vi "Teleop.vi"(10 "Match Info":T1={"Autonomous Elapsed Seconds"=0.0, "TeleOp Elapsed Seconds"=0.0, "Disabled Elapsed Seconds"=0.0, "Visited Autonomous"=FALSE, "Visited TeleOp"=FALSE, "Visited Disabled"=FALSE, "Autonomous Settings"={"Autonomous Style"=enum."Independent", "VI Refnum"=refnum}}, 11 "Call Context":T2) -> ()   [LabVIEW 2012]
doc: "This VI is called for each TeleOp packet received from the DS where the robot is not disabled. It is often used to read from the joysticks and update I/O or to update setpoints for timed control loops. It should complete and return within 20 milliseconds or it may miss DS packets."
uses:
  Robot Global Data.vi
  <vilib>/Rock Robotics/WPI/RobotDrive/WPI_RobotDriveMotorSelectorEnum.ctl
  <vilib>/Rock Robotics/WPI/Solenoid/WPI_SolenoidValue.ctl
  <vilib>/Rock Robotics/WPI/Solenoid/WPI_SolenoidSetEnum.vi
  <vilib>/Rock Robotics/WPI/RobotDrive/WPI_RobotDriveMecanumDrive_Cartesian.vi
  <vilib>/Rock Robotics/WPI/DriverStation/WPI_DriverStationMatch Info.ctl
  <vilib>/Rock Robotics/WPI/DriverStation/WPI_DriverStationDerivedRobotMode.ctl
panel:
  out "Frount/Rear drive speed":dbl=0.33
  out "MECH X/Y Speed":dbl=1.0
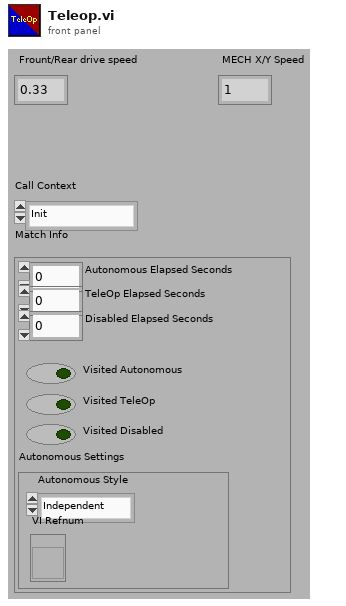
[diagram p1: front panel]
types:
  T1 = typedef "WPI_DriverStationMatch Info.ctl" = cluster{"Autonomous Elapsed Seconds":dbl, "TeleOp Elapsed Seconds":dbl, "Disabled Elapsed Seconds":dbl, "Visited Autonomous":bool, "Visited TeleOp":bool, "Visited Disabled":bool, "Autonomous Settings":cluster{"Autonomous Style":enum16{"Iterative", "Independent"}, "VI Refnum":refnum<vi>}}
  T2 = typedef "WPI_DriverStationDerivedRobotMode.ctl" = enum16{"Init", "Execute", "Stop"}
  T3 = typedef "WPI_SolenoidValue.ctl" = enum16{"Off", "On", "Forward", "Reverse"}
  T4 = typedef "WPI_JoystickDevRef.ctl" = cluster{"Device":T5}
  T5 = typedef "WPI_JoystickDeviceEnum.ctl" = enum16{"USB 1", "USB 2", "USB 3", "USB 4", "Kinect 1", "Kinect 2"}
  T6 = typedef "WPI_JoystickButtonState.ctl" = cluster{"Button 1":bool, "Button 2":bool, "Button 3":bool, "Button 4":bool, "Button 5":bool, "Button 6":bool, "Button 7":bool, "Button 8":bool, "Button 9":bool, "Button 10":bool, "Button 11":bool, "Button 12":bool}
  T7 = cluster{"axis 1 (x)":dbl, "axis 2 (y)":dbl, "axis 3 (throttle)":dbl, "axis 4":dbl, "axis 5":dbl, "axis 6":dbl}
  T8 = typedef "WPI_RobotDriveDevRef.ctl" = cluster{"DevStatus":errorcluster, "Motors[]":T9[], "Square Inputs":bool, "Max Output":dbl, "Isochronous":bool}
  T9 = typedef "WPI_MotorControlDeviceRef.ctl" = cluster{"DeviceStatus":errorcluster, "Type":enum16{"PWM", "CAN"}, "PWM":cluster{"Digital Module":T10, "PWM Channel":T11, "DeadBand":T12}, "CAN":cluster{"Device Number":u8, "Control Mode":T13, "Semaphore":T14, "Max Vout":dbl}, "Invert":bool, "TransformRef":T15, "InvTransformRef":T15}
  T10 = typedef "FPGA_TypedefDigitalModule.ctl" = enum16{"Digital Module 1", "Digital Module 2"}
  T11 = typedef "FPGA_DIOPWMChannel.ctl" = enum8{"PWM 1", "PWM 2", "PWM 3", "PWM 4", "PWM 5", "PWM 6", "PWM 7", "PWM 8", "PWM 9", "PWM 10", "Invalid"}
  T12 = typedef "WPI_PWMDeadband.ctl" = cluster{"Name":string, "maxPositivePwm":i32, "minPositivePwm":i32, "centerPwm":i32, "maxNegativePwm":i32, "minNegativePwm":i32, "angularRange":u16}
  T13 = typedef "WPI_CANJaguar_ControlMode.ctl" = enum8{"Percent VBus", "Current", "Speed", "Position", "Voltage"}
  T14 = typedef "Semaphore RefNum" = refnum<k1>
  T15 = typedef "WPI_PWMTransform_ConPane.ctl" = refnum<vi>
  T16 = typedef "WPI_RobotDriveMotorSelectorEnum.ctl" = enum16{"Rear Left Motor", "Rear Right Motor", "Front Left Motor", "Front Right Motor"}
  T17 = typedef "WPI_DigitalInputDevRef.ctl" = cluster{"DevStatus":errorcluster, "DIO Channel":T18, "Digital Module":T10}
  T18 = typedef "FPGA_DIOChannel.ctl" = enum8{"DIO 1", "DIO 2", "DIO 3", "DIO 4", "DIO 5", "DIO 6", "DIO 7", "DIO 8", "DIO 9", "DIO 10", "DIO 11", "DIO 12", "DIO 13", "DIO 14", "Invalid"}
  T19 = typedef "WPI_SolenoidDevRef.ctl" = cluster{"DevStatus":errorcluster, "Solenoid Module":T20, "Forward Solenoid Channel":T21, "Reverse Solenoid Channel":T21}
  T20 = typedef "FPGA_TypedefSolenoidModule.ctl" = enum16{"Solenoid Module 1", "Solenoid Module 2"}
  T21 = typedef "WPI_SolenoidChannel.ctl" = enum8{"Solenoid 1", "Solenoid 2", "Solenoid 3", "Solenoid 4", "Solenoid 5", "Solenoid 6", "Solenoid 7", "Solenoid 8", "Invalid"}
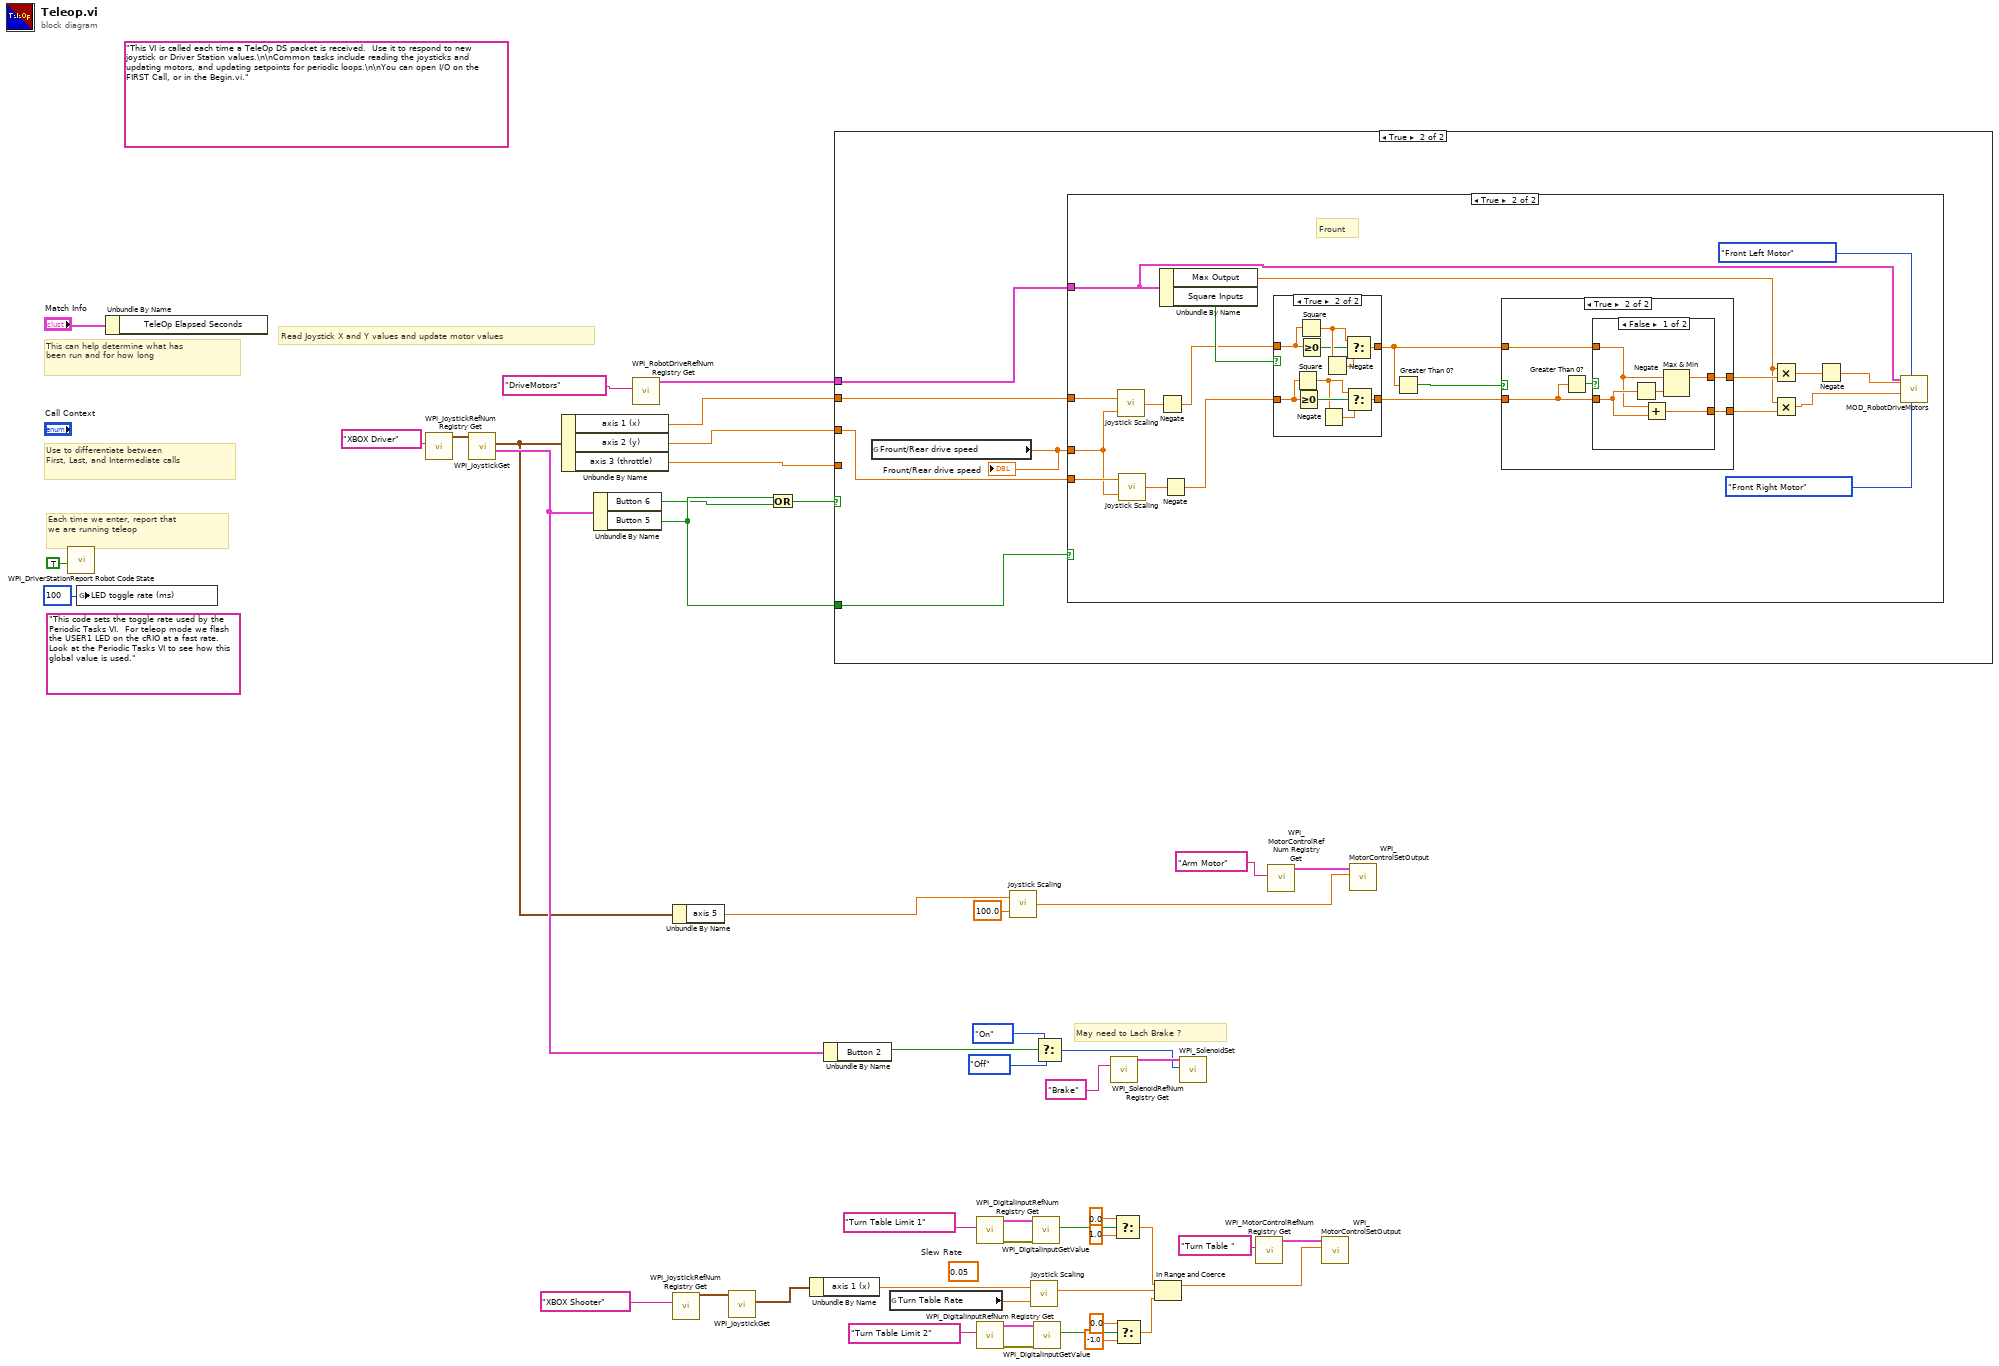
[diagram p0: block diagram]
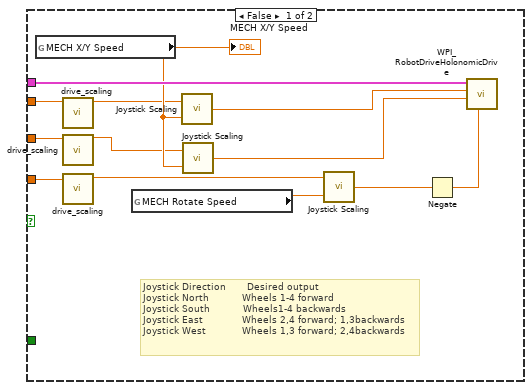
[diagram p2: hidden frame]
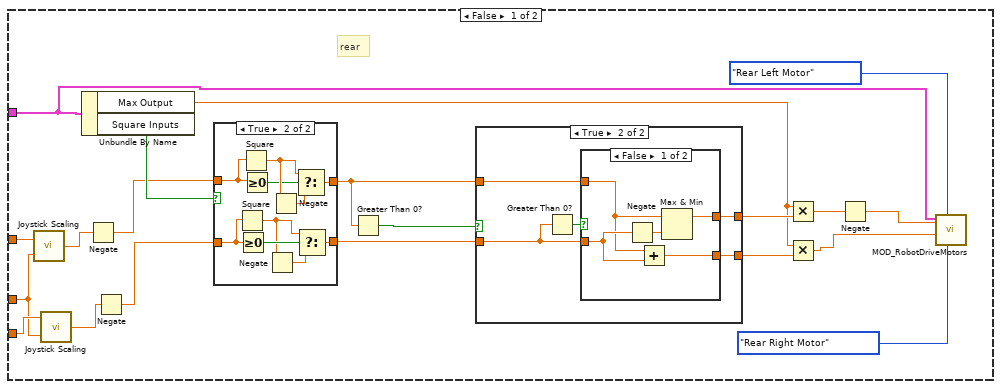
[diagram p3: hidden frame]
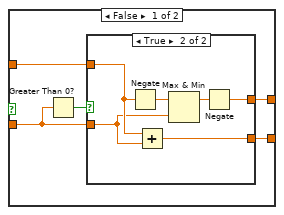
[diagram p4: hidden frame]
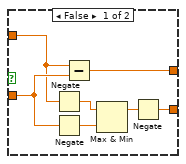
[diagram p5: hidden frame]
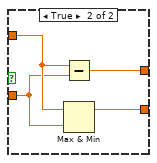
[diagram p6: hidden frame]
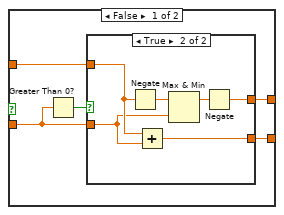
[diagram p8: hidden frame]
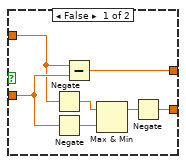
[diagram p9: hidden frame]
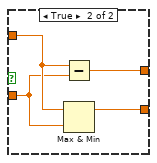
[diagram p10: hidden frame]
diagram:
  (unwired) 0.05  # Slew Rate
  (unwired) "This code sets the toggle rate used by the Periodic Tasks VI.  For teleop mode we flash the USER1 LED on the cRIO at a fast rate.  Look at the Periodic Tasks VI to see how this global value is used."
  (unwired) "This VI is called each time a TeleOp DS packet is received.  Use it to respond to new joystick or Driver Station values.\n\nCommon tasks include reading the joysticks and updating motors, and updating setpoints for periodic loops.\n\nYou can open I/O on the FIRST Call, or in the Begin.vi."
  # "May need to Lach Brake ?"
  # "Each time we enter, report that\nwe are running teleop"
  # "Use to differentiate between\nFirst, Last, and Intermediate calls"
  # "This can help determine what has\nbeen run and for how long"
  # "Read Joystick X and Y values and update motor values"
  n1 = call <vilib>:"WPI_DriverStationReport Robot Code State.vi"("TeleOp"=TRUE ("Autonomous")) -> ()  [unwired: 10 in, 1 out]
  n2 = global write "Robot Global Data.vi" "LED toggle rate (ms)"(u32 100 ("LED ms toggle rate")) -> ()
  n3 = Unbundle By Name("Match Info") -> ()  [unwired: 1 out]
  n4 = call <vilib>:"WPI_JoystickRefNum Registry Get.vi"("refnum name"="XBOX Driver") -> ("JoystickDevRef"=w47:T4)  [unwired: 1 in, 9 out]
  n5 = call <vilib>:"WPI_JoystickGet.vi"("JoystickDevRef"=w47) -> ("Buttons"=w8:T6, "Axes"=w7:T7)  [unwired: 1 in, 4 out]
  n6 = Unbundle By Name(w7) -> ("axis 1 (x)"=w43:dbl, "axis 2 (y)"=w44:dbl, "axis 3 (throttle)"=w41:dbl)
  n7 = Unbundle By Name(w8) -> ("Button 6"=w38:bool, "Button 5"=w39:bool)
  n8 = call <vilib>:"WPI_RobotDriveRefNum Registry Get.vi"("refnum name"="DriveMotors") -> ("RobotDriveDevRef"=w29:T8)  [unwired: 1 in, 9 out]
  n9 = Unbundle By Name(w7) -> ("axis 5"=w3:dbl)
  n10 = call <vilib>:"WPI_JoystickRefNum Registry Get.vi"("refnum name"="XBOX Shooter") -> ("JoystickDevRef"=w31:T4)  [unwired: 1 in, 9 out]
  n11 = call <vilib>:"WPI_JoystickGet.vi"("JoystickDevRef"=w31) -> ("Axes"=w30:T7)  [unwired: 1 in, 5 out]
  n12 = Or(x=w39, y=w38) -> (x .or. y?=w40:bool)
  n13 = Unbundle By Name(w30) -> ("axis 1 (x)"=w26:dbl)
  n14 = Unbundle By Name(w8) -> ("Button 2"=w33:bool)
  n15 = case shown="True" w40 {
    tunnel: w29 -> [w62 w65]
    tunnel: w44 -> [w52 w66]
    tunnel: w43 -> [w54 w67]
    tunnel: w41 -> [w58 _]
    tunnel: w39 -> [_ w64]
    frame False {
      # "Joystick Direction       Desired output\nJoystick North           Wheels 1-4 forward\nJoystick South           Wheels1-4 backwards\nJoystick East             Wheels 2,4 forward; 1,3backwards\nJoystick West            Wheels 1,3 forward; 2,4backwards"
      n16 = global read "Robot Global Data.vi" "MECH X/Y Speed"() -> (w59:dbl)
      "MECH X/Y Speed" <- w59
      n17 = call "drive_scaling.vi"("In"=w54) -> ("Out"=w55:dbl)  [unwired: 10 in]
      n18 = call "drive_scaling.vi"("In"=w52) -> ("Out"=w51:dbl)  [unwired: 10 in]
      n19 = call "drive_scaling.vi"("In"=w58) -> ("Out"=w57:dbl)  [unwired: 10 in]
      n20 = global read "Robot Global Data.vi" "MECH Rotate Speed"() -> (w60:dbl)
      n21 = call "Joystick Scaling.vi"("Scale (%)"=w59, "Input (+/- 1.00 volt)"=w55) -> ("Output"=w53:dbl)  [unwired: 1 in]
      n22 = call "Joystick Scaling.vi"("Scale (%)"=w59, "Input (+/- 1.00 volt)"=w51) -> ("Output"=w50:dbl)  [unwired: 1 in]
      n23 = call "Joystick Scaling.vi"("Scale (%)"=w60, "Input (+/- 1.00 volt)"=w57) -> ("Output"=w56:dbl)  [unwired: 1 in]
      n24 = Negate(x=w56) -> (-x=w61:dbl)
      n25 = call-poly <vilib>:"WPI_RobotDriveHolonomicDrive.vi"("Rotation"=w61, "Y"=w50, "X"=w53, "RobotDriveDevRef"=w62) -> ()  [unwired: 5 in, 3 out]
    }
    frame True {
      n26 = global read "Robot Global Data.vi" "Frount/Rear drive speed"() -> (w63:dbl)
      "Frount/Rear drive speed" <- w63
      n27 = case shown="True" w64 {
        tunnel: w63 -> [w68 w136]
        tunnel: w67 -> [w72 w137]
        tunnel: w66 -> [w69 w138]
        tunnel: w65 -> [w80 w139]
        frame False {
          # "rear"
          n28 = call "Joystick Scaling.vi"("Scale (%)"=w68, "Input (+/- 1.00 volt)"=w72) -> ("Output"=w71:dbl)  [unwired: 1 in]
          n29 = call "Joystick Scaling.vi"("Scale (%)"=w68, "Input (+/- 1.00 volt)"=w69) -> ("Output"=w70:dbl)  [unwired: 1 in]
          n30 = Unbundle By Name(w80) -> ("Max Output"=w81:dbl, "Square Inputs"=w87:bool)
          n31 = Negate(x=w71) -> (-x=w74:dbl)
          n32 = Negate(x=w70) -> (-x=w73:dbl)
          n33 = case shown="True" w87 {
            tunnel: [w120 w131] -> w84
            tunnel: [w121 w130] -> w85
            tunnel: w73 -> [w120 w129]
            tunnel: w74 -> [w121 w128]
            frame False {
            }
            frame True {
              n34 = Square(x=w129) -> (x^2=w126:dbl)
              n35 = Greater Or Equal To 0?(x=w129) -> (x >= 0?=w127:bool)
              n36 = Square(x=w128) -> (x^2=w123:dbl)
              n37 = Greater Or Equal To 0?(x=w128) -> (x >= 0?=w122:bool)
              n38 = Negate(x=w126) -> (-x=w125:dbl)
              n39 = Negate(x=w123) -> (-x=w124:dbl)
              n40 = Select(t=w123, s=w122, f=w124) -> (s? t:f=w130:dbl)
              n41 = Select(t=w126, s=w127, f=w125) -> (s? t:f=w131:dbl)
            }
          }
          n42 = Greater Than 0?(x=w85) -> (x > 0?=w86:bool)
          n43 = case shown="True" w86 {
            tunnel: w84 -> [w91 w109]
            tunnel: w85 -> [w90 w108]
            tunnel: [w89 w107] -> w83
            tunnel: [w88 w106] -> w82
            frame False {
              n44 = Greater Than 0?(x=w91) -> (x > 0?=w92:bool)
              n45 = case shown="True" w92 {
                tunnel: w91 -> [w99 w101]
                tunnel: w90 -> [w97 w102]
                tunnel: [w93 w103] -> w89
                tunnel: [w94 w100] -> w88
                frame False {
                  n46 = Negate(x=w97) -> (-x=w98:dbl)
                  n47 = Negate(x=w99) -> (-x=w96:dbl)
                  n48 = Subtract(x=w97, y=w99) -> (x-y=w93:dbl)
                  n49 = Max & Min(x=w98, y=w96) -> (max(x,y)=w95:dbl)  [unwired: 1 out]
                  n50 = Negate(x=w95) -> (-x=w94:dbl)
                }
                frame True {
                  n51 = Negate(x=w102) -> (-x=w105:dbl)
                  n52 = Add(x=w102, y=w101) -> (x+y=w100:dbl)
                  n53 = Max & Min(x=w105, y=w101) -> (max(x,y)=w104:dbl)  [unwired: 1 out]
                  n54 = Negate(x=w104) -> (-x=w103:dbl)
                }
              }
            }
            frame True {
              n55 = Greater Than 0?(x=w109) -> (x > 0?=w110:bool)
              n56 = case shown="False" w110 {
                tunnel: w109 -> [w115 w117]
                tunnel: w108 -> [w112 w118]
                tunnel: [w113 w116] -> w107
                tunnel: [w111 w119] -> w106
                frame False {
                  n57 = Negate(x=w115) -> (-x=w114:dbl)
                  n58 = Add(x=w112, y=w115) -> (x+y=w111:dbl)
                  n59 = Max & Min(x=w112, y=w114) -> (max(x,y)=w113:dbl)  [unwired: 1 out]
                }
                frame True {
                  n60 = Subtract(x=w118, y=w117) -> (x-y=w116:dbl)
                  n61 = Max & Min(x=w118, y=w117) -> (max(x,y)=w119:dbl)  [unwired: 1 out]
                }
              }
            }
          }
          n62 = Multiply(x=w81, y=w83) -> (x*y=w79:dbl)
          n63 = Multiply(x=w81, y=w82) -> (x*y=w78:dbl)
          n64 = Negate(x=w79) -> (-x=w75:dbl)
          n65 = call "MOD_RobotDriveMotors.vi"("MotorIndex 2"=WPI_RobotDriveMotorSelectorEnum."Rear Right Motor", "MotorIndex"=WPI_RobotDriveMotorSelectorEnum."Rear Left Motor", "RightSpeed"=w78, "LeftSpeed"=w75, "RobotDriveDevRef"=w80) -> ()  [unwired: 5 in, 2 out]
        }
        frame True {
          # "Frount"
          n66 = call "Joystick Scaling.vi"("Scale (%)"=w136, "Input (+/- 1.00 volt)"=w137) -> ("Output"=w135:dbl)  [unwired: 1 in]
          n67 = call "Joystick Scaling.vi"("Scale (%)"=w136, "Input (+/- 1.00 volt)"=w138) -> ("Output"=w134:dbl)  [unwired: 1 in]
          n68 = Negate(x=w135) -> (-x=w133:dbl)
          n69 = Unbundle By Name(w139) -> ("Max Output"=w145:dbl, "Square Inputs"=w151:bool)
          n70 = Negate(x=w134) -> (-x=w132:dbl)
          n71 = case shown="True" w151 {
            tunnel: [w184 w195] -> w148
            tunnel: [w185 w194] -> w149
            tunnel: w132 -> [w184 w193]
            tunnel: w133 -> [w185 w192]
            frame False {
            }
            frame True {
              n72 = Square(x=w193) -> (x^2=w190:dbl)
              n73 = Greater Or Equal To 0?(x=w193) -> (x >= 0?=w191:bool)
              n74 = Square(x=w192) -> (x^2=w187:dbl)
              n75 = Greater Or Equal To 0?(x=w192) -> (x >= 0?=w186:bool)
              n76 = Negate(x=w190) -> (-x=w189:dbl)
              n77 = Negate(x=w187) -> (-x=w188:dbl)
              n78 = Select(t=w187, s=w186, f=w188) -> (s? t:f=w194:dbl)
              n79 = Select(t=w190, s=w191, f=w189) -> (s? t:f=w195:dbl)
            }
          }
          n80 = Greater Than 0?(x=w149) -> (x > 0?=w150:bool)
          n81 = case shown="True" w150 {
            tunnel: w148 -> [w155 w173]
            tunnel: w149 -> [w154 w172]
            tunnel: [w153 w171] -> w147
            tunnel: [w152 w170] -> w146
            frame False {
              n82 = Greater Than 0?(x=w155) -> (x > 0?=w156:bool)
              n83 = case shown="True" w156 {
                tunnel: w155 -> [w163 w165]
                tunnel: w154 -> [w161 w166]
                tunnel: [w157 w167] -> w153
                tunnel: [w158 w164] -> w152
                frame False {
                  n84 = Negate(x=w161) -> (-x=w162:dbl)
                  n85 = Negate(x=w163) -> (-x=w160:dbl)
                  n86 = Subtract(x=w161, y=w163) -> (x-y=w157:dbl)
                  n87 = Max & Min(x=w162, y=w160) -> (max(x,y)=w159:dbl)  [unwired: 1 out]
                  n88 = Negate(x=w159) -> (-x=w158:dbl)
                }
                frame True {
                  n89 = Negate(x=w166) -> (-x=w169:dbl)
                  n90 = Add(x=w166, y=w165) -> (x+y=w164:dbl)
                  n91 = Max & Min(x=w169, y=w165) -> (max(x,y)=w168:dbl)  [unwired: 1 out]
                  n92 = Negate(x=w168) -> (-x=w167:dbl)
                }
              }
            }
            frame True {
              n93 = Greater Than 0?(x=w173) -> (x > 0?=w174:bool)
              n94 = case shown="False" w174 {
                tunnel: w173 -> [w179 w181]
                tunnel: w172 -> [w176 w182]
                tunnel: [w177 w180] -> w171
                tunnel: [w175 w183] -> w170
                frame False {
                  n95 = Negate(x=w179) -> (-x=w178:dbl)
                  n96 = Add(x=w176, y=w179) -> (x+y=w175:dbl)
                  n97 = Max & Min(x=w176, y=w178) -> (max(x,y)=w177:dbl)  [unwired: 1 out]
                }
                frame True {
                  n98 = Subtract(x=w182, y=w181) -> (x-y=w180:dbl)
                  n99 = Max & Min(x=w182, y=w181) -> (max(x,y)=w183:dbl)  [unwired: 1 out]
                }
              }
            }
          }
          n100 = Multiply(x=w145, y=w147) -> (x*y=w144:dbl)
          n101 = Multiply(x=w145, y=w146) -> (x*y=w143:dbl)
          n102 = Negate(x=w144) -> (-x=w140:dbl)
          n103 = call "MOD_RobotDriveMotors.vi"("MotorIndex 2"=WPI_RobotDriveMotorSelectorEnum."Front Right Motor", "MotorIndex"=WPI_RobotDriveMotorSelectorEnum."Front Left Motor", "RightSpeed"=w143, "LeftSpeed"=w140, "RobotDriveDevRef"=w139) -> ()  [unwired: 5 in, 2 out]
        }
      }
    }
  }
  n104 = global read "Robot Global Data.vi" "Turn Table Rate"() -> (w25:dbl)
  n105 = call <vilib>:"WPI_DigitalInputRefNum Registry Get.vi"("refnum name"="Turn Table Limit 1") -> ("error out"=w23:errorcluster, "DigitalInputDevRef"=w22:T17)  [unwired: 9 in]
  n106 = call <vilib>:"WPI_DigitalInputRefNum Registry Get.vi"("refnum name"="Turn Table Limit 2") -> ("error out"=w16:errorcluster, "DigitalInputDevRef"=w17:T17)  [unwired: 9 in]
  n107 = call "Joystick Scaling.vi"("Scale (%)"=100.0, "Input (+/- 1.00 volt)"=w3) -> ("Output"=w1:dbl)  [unwired: 1 in]
  n108 = call "Joystick Scaling.vi"("Scale (%)"=w25, "Input (+/- 1.00 volt)"=w26) -> ("Output"=w11:dbl)  [unwired: 1 in]
  n109 = call <vilib>:"WPI_DigitalInputGetValue.vi"("error in (no error)"=w23, "DigitalInputDevRef"=w22) -> ("Value"=w10:bool)  [unwired: 7 in, 2 out]
  n110 = call <vilib>:"WPI_DigitalInputGetValue.vi"("error in (no error)"=w16, "DigitalInputDevRef"=w17) -> ("Value"=w9:bool)  [unwired: 7 in, 2 out]
  n111 = Select(t=WPI_SolenoidValue."On" ("Value"), s=w33, f=WPI_SolenoidValue."Off" ("Value")) -> (s? t:f=w35:T3)
  n112 = call <vilib>:"WPI_SolenoidRefNum Registry Get.vi"("refnum name"="Brake") -> ("SolenoidDevRef"=w37:T19)  [unwired: 9 in, 1 out]
  n113 = Select(t=0.0, s=w10, f=1.0) -> (s? t:f=w14:dbl)
  n114 = Select(t=0.0, s=w9, f=-1.0) -> (s? t:f=w13:dbl)
  n115 = In Range and Coerce(upper limit=w14, x=w11, lower limit=w13) -> (coerced(x)=w12:dbl)  [unwired: 1 out]
  n116 = call-poly <vilib>:"WPI_SolenoidSet.vi"("Value"=w35, "SolenoidDevRef"=w37) -> ()  [unwired: 8 in, 2 out]
  n117 = call <vilib>:"WPI_MotorControlRefNum Registry Get.vi"("refnum name"="Turn Table ") -> ("MotorControlDevRef"=w28:T9)  [unwired: 9 in, 1 out]
  n118 = call <vilib>:"WPI_MotorControlRefNum Registry Get.vi"("refnum name"="Arm Motor") -> ("MotorControlDevRef"=w5:T9)  [unwired: 9 in, 1 out]
  n119 = call <vilib>:"WPI_MotorControlSetOutput.vi"("Output"=w12, "MotorControlDevRef"=w28) -> ()  [unwired: 7 in, 3 out]
  n120 = call <vilib>:"WPI_MotorControlSetOutput.vi"("Output"=w1, "MotorControlDevRef"=w5) -> ()  [unwired: 7 in, 3 out]
